vi "Get FPGA Reference.vi"(8 "Error In":errorcluster, 11 "Audio Analyzer In":refnum<class "Audio Analyzer.lvclass">) -> (0 "Error Out":errorcluster, 2 "FPGA Reference":T1, 3 "Audio Analyzer Out":refnum<class "Audio Analyzer.lvclass">)   [LabVIEW 2021, in "Audio Analyzer.lvclass"]
uses:
  Audio Analyzer.lvclass
  Public/Controls/FPGA Reference.ctl
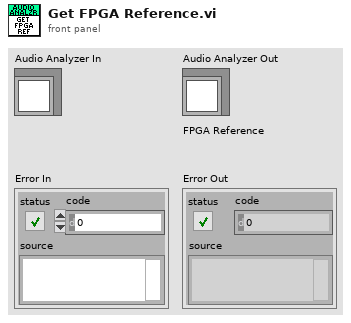
[diagram p1: front panel]
types:
  T1 = typedef "Audio Analyzer.lvclass/FPGA Reference.ctl" = refnum<k20>
  T2 = typedef "Audio Analyzer.lvclass/Data.ctl" = cluster{"Audio Spectrum Notifier":refnum<notifier>, "FPGA Reference":T1}
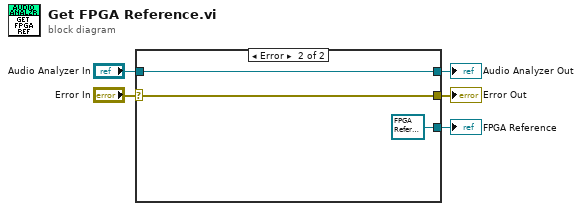
[diagram p0: block diagram]
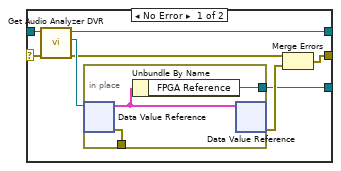
[diagram p2: hidden frame]
diagram:
  n1 = case shown="Error" "Error In" {
    selector: "Error In" -> [w10 w18]
    tunnel: [w12 w18] -> w2
    tunnel: [w9 w19] -> w4
    tunnel: "Audio Analyzer In" -> [w11 w19]
    tunnel: [w6 T1 refnum ("FPGA Reference")] -> w1
    frame No Error {
      n2 = call "Get Audio Analyzer DVR.vi"("Error In"=w10, "Audio Analyzer In"=w11) -> ("Error Out"=w7:errorcluster, "DVR"=w8:refnum<data-value>, "Audio Analyzer Out"=w9:refnum<class "Audio Analyzer.lvclass">)  [unwired: 7 in]
      n3 = in-place {
        in-place-border: [w14] -> w6
        in-place-border: [w16] -> _
        n4 = in-place-dvr #1(w8) -> (w15:T2, w16:errorcluster)
        n5 = Unbundle By Name(w15) -> ("FPGA Reference"=w14:T1)
        n6 = in-place-dvr #1(w15) -> (w13:errorcluster)  [unwired: 1 out]
      }
      n7 = Merge Errors(w7, w13) -> (w12:errorcluster)
    }
    frame Error {
    }
  }
  "Audio Analyzer Out" <- w4
  "Error Out" <- w2
  "FPGA Reference" <- w1
